vi "GrabSingleImage.vi"() -> (3 "Image Pixels (U8)":u8[][](array[numeric]))   [LabVIEW 2011]
uses:
  CmdData_NewFrame.ctl
  <vilib>/vision/Image Controls.llb/IMAQ Image.ctl
  CmdEnum_CameraFrameType.ctl
  CmdData_GrabParams.ctl
  qtrk/QTrk.llb/QTrkInstance.ctl
  CmdEnum_CameraIn.ctl
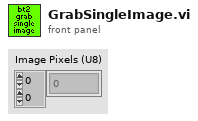
[diagram p1: front panel]
types:
  T1 = typedef "CmdData_NewFrame.ctl" = cluster{"Buffer Image":T2, "Frame #":i32, "Hardware ROI Index":i32, "Timestamp":dbl, "Type":T3}
  T2 = typedef "IMAQ Image.ctl" = refnum<image>
  T3 = typedef "CmdEnum_CameraFrameType.ctl" = enum16{"Full", "HardwareROI", "EndGrabMarker"}
  T4 = typedef "CmdData_GrabParams.ctl" = cluster{"QTrk Instance":T5, "Output Queue":refnum<queue>}
  T5 = typedef "QTrkInstance.ctl" = cluster{"QTrk Pointer":u64}
  T6 = typedef "CmdEnum_CameraIn.ctl" = enum32{"Init", "Close", "ShowSettingsDialog", "EndGrab", "GrabZLUT", "GrabToTracker", "GrabToQueue", "AdjustROIs"}
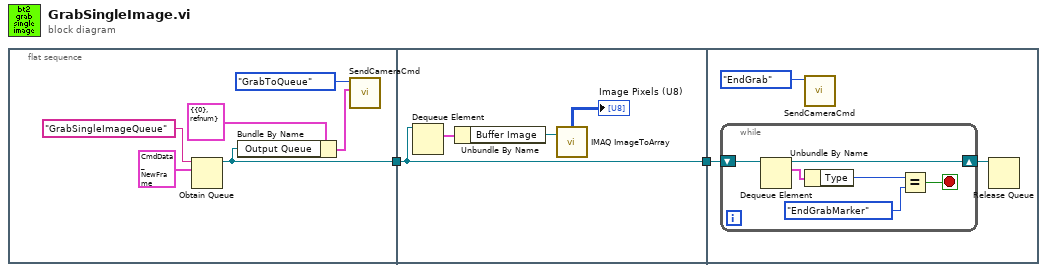
[diagram p0: block diagram]
diagram:
  n1 = flat-sequence {
    tunnel: [w3] -> w2
    tunnel: w2 -> [w9]
    tunnel: [w9] -> w1
    tunnel: w1 -> [w14]
    frame #0 {
      n2 = Obtain Queue(name (unnamed)="GrabSingleImageQueue", element data type=T1 {"Buffer Image"=refnum, "Frame #"=0, "Hardware ROI Index"=0, "Timestamp"=0.0, "Type"=enum."Full"} ("Cluster")) -> (queue out=w3:refnum<queue>)  [unwired: 3 in, 2 out]
      n3 = Bundle By Name(cluster=T4 {"QTrk Instance"={"QTrk Pointer"=0}, "Output Queue"=refnum} ("GrabToTrackerParameters"), "Output Queue"=w3) -> (w4:T4)
      n4 = call "SendCameraCmd.vi"("Msg Data"=w4, "Camera cmd (SettingsDlg)"=CmdEnum_CameraIn."GrabToQueue") -> ()  [unwired: 10 in]
    }
    frame #1 {
      n5 = Dequeue Element(queue=w9) -> (element=w11:T1)  [unwired: 2 in, 3 out]
      n6 = Unbundle By Name(w11) -> ("Buffer Image"=w12:T2)
      n7 = call "IMAQ ImageToArray"("Image"=w12) -> ("Image Pixels (U8)"=→"Image Pixels (U8)":u8[][])  [unwired: 3 in, 4 out]
    }
    frame #2 {
      n8 = while {
        shift-right: [w17] -> w13
        shift-left: w14 -> [w16]
        stop <- w18 stop-if-true
        n9 = Dequeue Element(queue=w16) -> (queue out=w17:refnum<queue>, element=w21:T1)  [unwired: 2 in, 2 out]
        n10 = Unbundle By Name(w21) -> ("Type"=w20:T3)
        n11 = Equal?(x=w20, y=CmdEnum_CameraFrameType."EndGrabMarker") -> (x = y?=w18:bool)
      }
      n12 = call "SendCameraCmd.vi"("Camera cmd (SettingsDlg)"=CmdEnum_CameraIn."EndGrab") -> ()  [unwired: 11 in]
      n13 = Release Queue(queue=w13) -> ()  [unwired: 2 in, 3 out]
    }
  }
